vi "GetAllFiles.vi"(8 "error in (no error)":errorcluster, 10 "Dest Folder":path, 11 "Local Folder":path) -> (0 "error out":errorcluster, 2 "Dest Files":path[](array[path]), 3 "Local Files":path[](array[path]))   [LabVIEW 2022 SP3]
panel:
  out "Dest Count":i32
  out "Local Count":i32
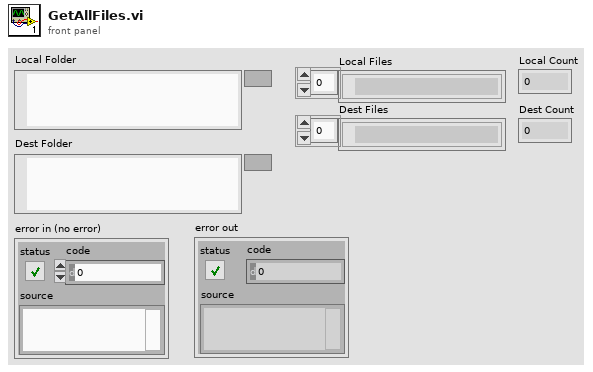
[diagram p1: front panel]
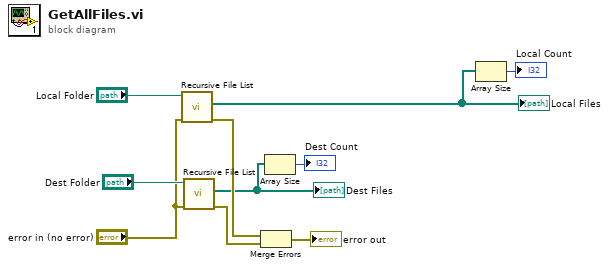
[diagram p0: block diagram]
diagram:
  n1 = call <vilib>:"Recursive File List.vi"("error in (no error)"="error in (no error)", "Folder Path"="Local Folder") -> ("error out"=w7:errorcluster, "All Files in Dir"=w4:path[])  [unwired: 5 in, 3 out]
  "Local Files" <- w4
  n2 = call <vilib>:"Recursive File List.vi"("error in (no error)"="error in (no error)", "Folder Path"="Dest Folder") -> ("error out"=w6:errorcluster, "All Files in Dir"=w2:path[])  [unwired: 5 in, 3 out]
  "Dest Files" <- w2
  n3 = Merge Errors(w7, w6) -> (→"error out":errorcluster)
  n4 = Array Size(array=w2) -> (size(s)=→"Dest Count":i32)
  n5 = Array Size(array=w4) -> (size(s)=→"Local Count":i32)
